vi "Boolean Array Test.vi"() -> ()   [LabVIEW 2021]
uses:
  Source/Omni-Bus/Omni_Bus.lvclass
  Source/Omni-Bus/Support/Broad Types.ctl
  Source/Local Bus/Local Bus.lvclass
  <vilib>/Utility/Data Type/Type Definitions/Data Type.ctl
  <vilib>/Utility/Data Type/NI_Data Type.lvlib
  C:/Users/Tim/Documents/GitHub/Omni-Bus/Source/Omni-Bus/Bus Access/Bus_Access.lvclass
panel:
  in  "Array":bool[](array[boolean])
  out "Booleans":bool[](array[boolean])
  out "error out 3":errorcluster
  out "error out 2":errorcluster
  in  "Tag 2":string[](array[string])
  in  "stop":bool
  in  "Tags":string[](array[string])
  out "error out":errorcluster
  out "Tags":string[](array[string])
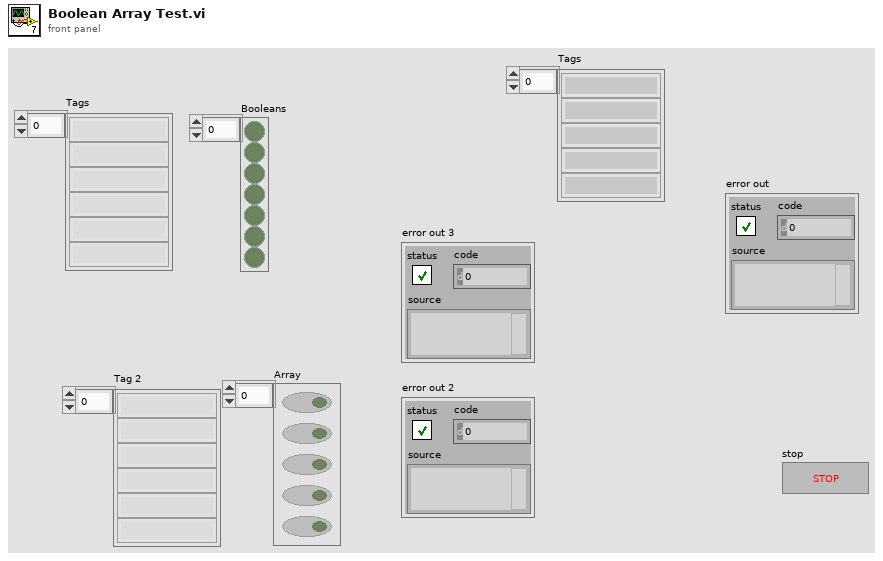
[diagram p1: front panel]
types:
  T1 = typedef "NI_Data Type.lvlib/Data Type.ctl" = enum8{"Invalid Type", "Void", "I8", "I16", "I32", "I64", "U8", "U16", "U32", "U64", "Single Float", "Double Float", "Extended Float", "Single Complex", "Double Complex", "Extended Complex", "Enum U8", "Enum U16", "Enum U32", "Enum U64", "Single Float With Unit", "Double Float With Unit", "Extended Float With Unit", "Single Complex with Unit", "Double Complex with Unit", "Extended Complex with Unit", "Boolean", "String", "Path", "Picture", "Tag", "Array", "Cluster", "Variant", "LV Variant", "Waveform", "Timestamp", "Digital Waveform", "Digital Data", "ExpressData", "Refnum", "External Data", "VI", "Poly VI", "LabVIEW Class Instance", "Fixed Point", "Set Collection", "Map Collection"}
  T2 = typedef "Omni_Bus.lvclass/Broad Types.ctl" = enum16{"All Tags", "NI Specific Type", "Boolean", "String", "Numeric", "Float", "Integer", "Collection", "All Value Types", "Non Value Types"}
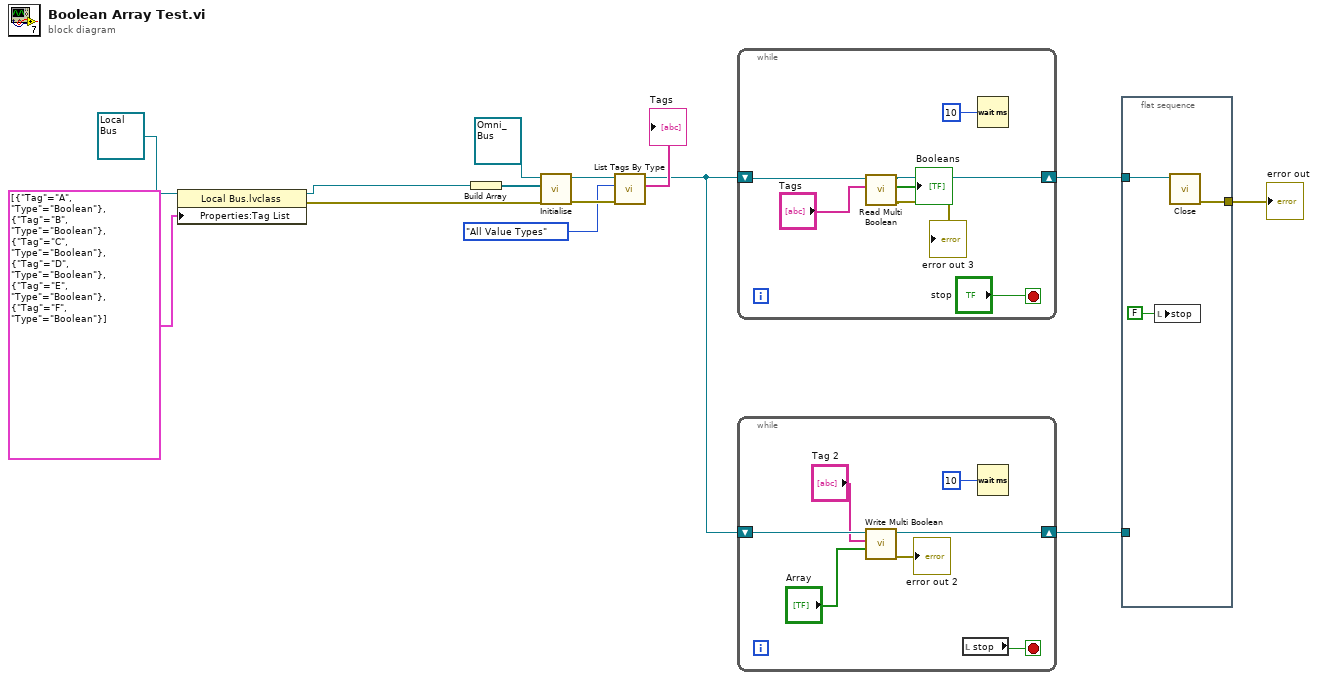
[diagram p0: block diagram]
diagram:
  n1 = property class="Local Bus.lvclass"(reference=refnum<class "Local Bus.lvclass"> refnum ("Local Bus.lvclass"), "Properties:Tag List"=cluster{"Tag":string, "Type":T1}[] [{"Tag"="A", "Type"=enum."Boolean"}, {"Tag"="B", "Type"=enum."Boolean"}, {"Tag"="C", "Type"=enum."Boolean"}, {"Tag"="D", "Type"=enum."Boolean"}, {"Tag"="E", "Type"=enum."Boolean"}, {"Tag"="F", "Type"=enum."Boolean"}] ("Tag List")) -> (reference out=w7:refnum<class "Local Bus.lvclass">, error out=w6:errorcluster)  [unwired: 1 in]
  n2 = Build Array(w7) -> (w13:refnum<class "Local Bus.lvclass">[])
  n3 = call-dynamic "Initialise.vi"("error in (no error)"=w6, "Bus Access"=w13, "Var Bus in"=refnum<class "Omni_Bus.lvclass"> refnum) -> ("error out"=w11:errorcluster, "Var Bus out"=w12:refnum<class "Omni_Bus.lvclass">)  [unwired: 7 in]
  n4 = call-dynamic "List Tags By Type.vi"("error in (no error)"=w11, "Broad Types"=Broad_Types."All Value Types", "Var Bus in"=w12) -> ("Tags"=→"Tags":string[], "Var Bus out"=w2:refnum<class "Omni_Bus.lvclass">)  [unwired: 5 in, 2 out]
  n5 = while {
    shift-right: [w19] -> w3
    shift-left: w2 -> [w18]
    stop <- "stop" stop-if-true
    n6 = call "Read Multi Boolean.vi"("Tags"="Tags", "Var Bus in"=w18) -> ("error out"=→"error out 3":errorcluster, "Booleans"=→"Booleans":bool[], "Var Bus out"=w19:refnum<class "Omni_Bus.lvclass">)  [unwired: 7 in]
    n7 = Wait (ms)(milliseconds to wait=u32 10) -> ()  [unwired: 1 out]
  }
  n8 = while {
    shift-right: [w25] -> w1
    shift-left: w2 -> [w26]
    stop <- w28 stop-if-true
    n9 = call "Write Multi Boolean.vi"("Array"="Array", "Tag"="Tag 2", "Omni_Bus in"=w26) -> ("error out"=→"error out 2":errorcluster, "Omni_Bus out"=w25:refnum<class "Omni_Bus.lvclass">)  [unwired: 7 in]
    n10 = local read "stop"() -> (w28:bool)
    n11 = Wait (ms)(milliseconds to wait=u32 10) -> ()  [unwired: 1 out]
  }
  n12 = flat-sequence {
    tunnel: [w31] -> w8
    tunnel: w3 -> [w30]
    tunnel: w1 -> [_]
    frame #0 {
      n13 = local write "stop"(FALSE ("stop")) -> ()
      n14 = call-dynamic "Close.vi"("Data in"=w30) -> ("error out"=w31:errorcluster)  [unwired: 9 in, 1 out]
    }
  }
  "error out" <- w8
